vi "Obtain.vi"(8 "error in (no error)":errorcluster) -> (0 "error out":errorcluster, 3 "LV Argument Parser out":refnum<class "LV Argument Parser.lvclass">)   [LabVIEW 2020, in "LV ArgParse.lvlib" / "LV Argument Parser.lvclass"]
uses:
  LV Argument Parser.lvclass
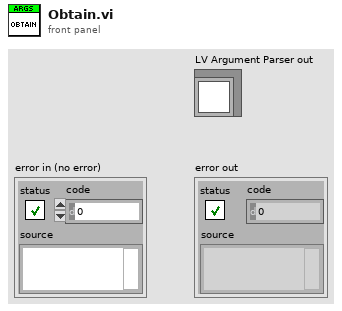
[diagram p1: front panel]
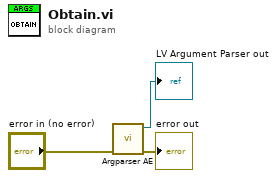
[diagram p0: block diagram]
diagram:
  n1 = call "Argparser AE.vi"("error in (no error)"="error in (no error)") -> ("error out"=→"error out":errorcluster, "LV Argument Parser out"=→"LV Argument Parser out":refnum<class "LV Argument Parser.lvclass">)  [unwired: 9 in]
